vi "Set Carrier Phase.vi"(0 "Session Handle in":T1, 5 "Phase":dbl, 11 "error in (no error)":errorcluster) -> (4 "Session Handle out":T1, 6 "Error Code":string, 15 "error out":errorcluster)   [LabVIEW 2015, in "PAS.lvclass"]
uses:
  PAS.lvclass
  Typedefs/Session Handle.ctl
panel:
  out "Success?":bool
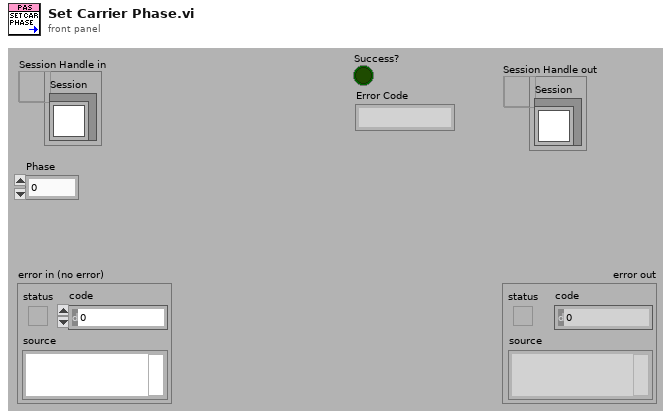
[diagram p1: front panel]
types:
  T1 = typedef "PAS.lvclass/Session Handle.ctl" = refnum<data-value>
  T2 = typedef "XNET Frame CAN.ctl" = cluster{"timestamp":timestamp, "payload":u8[], "identifier":u32, "type":T3, "extended?":bool, "echo?":bool}
  T3 = typedef "XNET Frame Type CAN.ctl" = u8
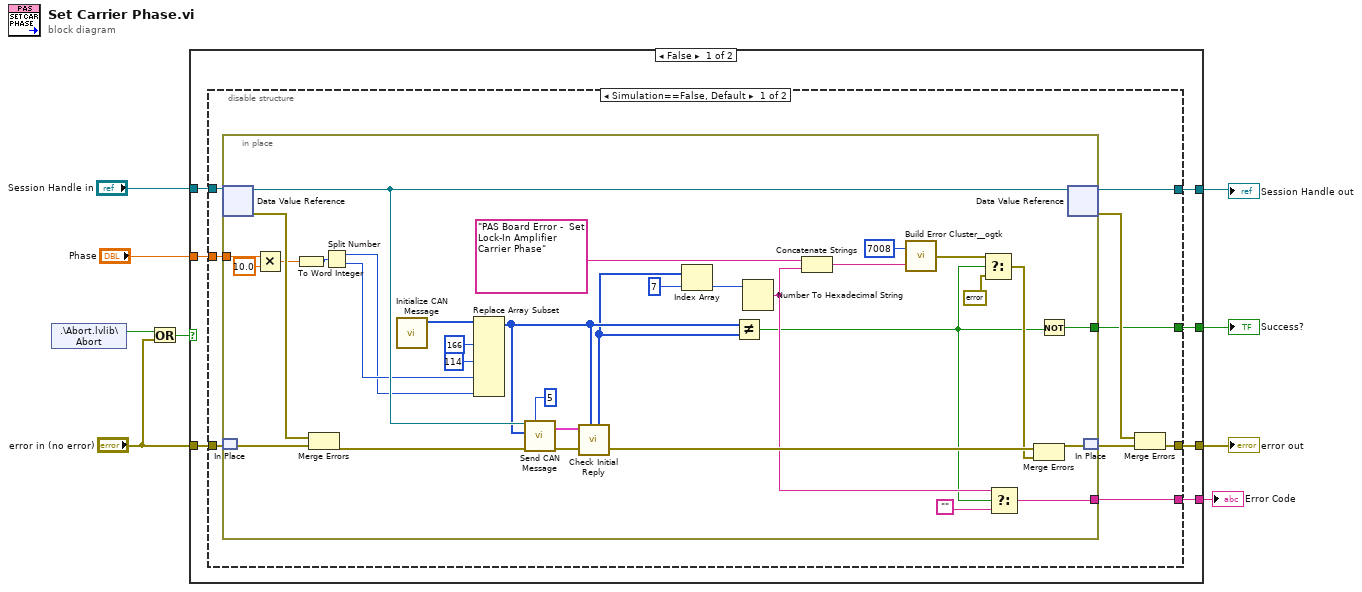
[diagram p0: block diagram]
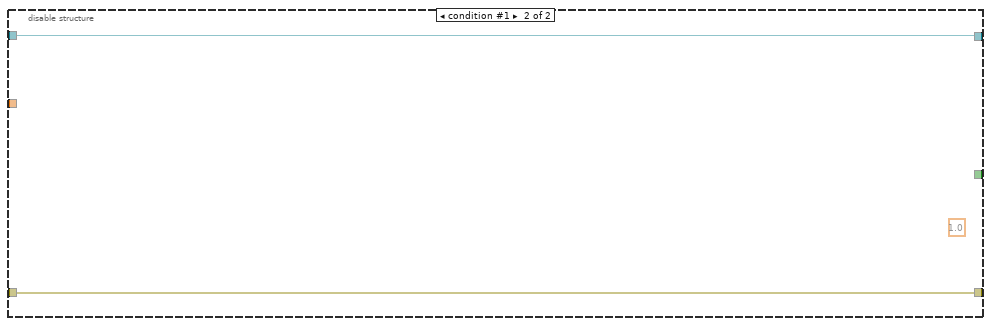
[diagram p2: hidden frame]
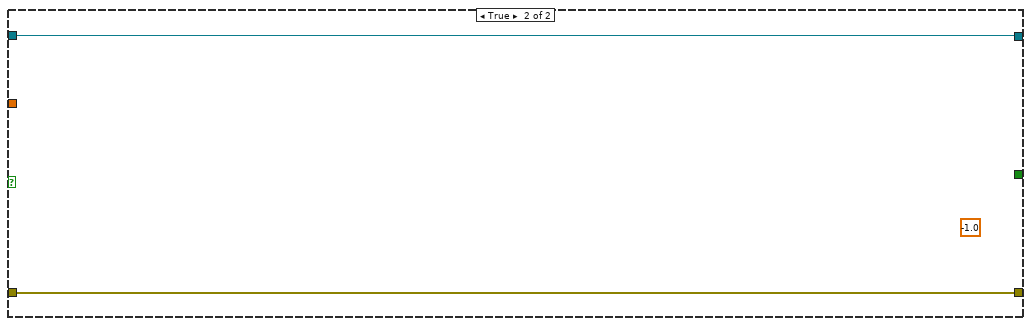
[diagram p3: hidden frame]
diagram:
  n1 = shared-variable ".\\Abort.lvlib\\Abort"() -> (w6:bool)  [unwired: 1 in, 1 out]
  n2 = Or(x=w6, y="error in (no error)") -> (x .or. y?=w4:bool)
  n3 = case shown="False" w4 {
    tunnel: [w16 w61] -> w8
    tunnel: [w15 w60] -> w7
    tunnel: "Session Handle in" -> [w14 w61]
    tunnel: "error in (no error)" -> [w13 w60]
    tunnel: [w12 _] -> w3
    tunnel: "Phase" -> [w11 _]
    tunnel: [w10 _] -> w1
    frame False {
      n4 = disable-structure shown="Simulation==False, Default" {
        disable-tunnel: [w25 w59] -> w16
        disable-tunnel: [w22 w58] -> w15
        disable-tunnel: w14 -> [w21 w59]
        disable-tunnel: w13 -> [w20 w58]
        disable-tunnel: [w19 _] -> w12
        disable-tunnel: w11 -> [w18 _]
        disable-tunnel: [w17 _] -> w10
        frame condition #0 (active) {
          n5 = in-place {
            in-place-border: [w47] -> w19
            in-place-border: w18 -> [w38]
            in-place-border: [w26] -> w17
            n6 = in-place-dvr #1(w21) -> (w50:refnum<class "PAS.lvclass">, w54:errorcluster)
            n7 = in-place-match #2(w20) -> (w53:errorcluster)
            n8 = Multiply(x=w38, y=10.0) -> (x*y=w36:dbl)
            n9 = To Word Integer(number=w36) -> (16bit integer=w41:i16)
            n10 = Merge Errors(w54, w53) -> (w49:errorcluster)
            n11 = Split Number(x=w41) -> (hi(x)=w39:u8, lo(x)=w40:u8)
            n12 = call "Initialize CAN Message.vi"() -> ("Initial Payload"=w55:u8[])  [unwired: 11 in]
            n13 = Replace Array Subset(array=w55, new element #1=u8 166 ("new element/subarray"), new element #2=u8 114 ("new element/subarray"), new element #3=w40, new element #4=w39) -> (w35:u8[])  [unwired: 4 in]
            n14 = call "Send CAN Message.vi"("Number of Retries"=5, "error in (no error)"=w49, "payload"=w35, "Gas In"=w50) -> ("error out"=w43:errorcluster, "Reply"=w51:T2[])  [unwired: 5 in, 1 out]
            n15 = call "Check Initial Reply.vi"("Write Message"=w35, "Reply"=w51) -> ("Whole Payload"=w31:u8[])  [unwired: 7 in, 2 out]
            n16 = Index Array(array=w31, index=7) -> (element=w33:u8)
            n17 = Not Equal?(x=w35, y=w31) -> (x != y?=w27:bool)
            n18 = Number To Hexadecimal String(2:w33) -> (0:w28:string)  [unwired: 1 in]
            n19 = Concatenate Strings("PAS Board Error -  Set Lock-In Amplifier Carrier Phase" ("string"), w28) -> (w32:string)
            n20 = call <userlib>:"Build Error Cluster__ogtk.vi"("String to Prepend to source (\"\")"=w32, "code"=7008) -> ("error out"=w46:errorcluster)
            n21 = Select(t=w46, s=w27, f=errorcluster {"status"=FALSE, "code"=0, "source"=""}) -> (s? t:f=w42:errorcluster)
            n22 = Select(t=w28, s=w27, f="") -> (s? t:f=w26:string)
            n23 = Merge Errors(w43, w42) -> (w56:errorcluster)
            n24 = Not(x=w27) -> (.not. x?=w47:bool)
            n25 = in-place-dvr #1(w50) -> (w25:T1, w23:errorcluster)
            n26 = in-place-match #2(w56) -> (w24:errorcluster)
          }
          n27 = Merge Errors(w23, w24) -> (w22:errorcluster)
        }
        frame condition #1 {
          (unwired) 1.0
        }
      }
    }
    frame True {
      (unwired) -1.0
    }
  }
  "Session Handle out" <- w8
  "error out" <- w7
  "Success?" <- w3
  "Error Code" <- w1
